vi "Create Bucket.vi"(7 "Request parameters":T1, 8 "error in (no error)":errorcluster, 9 "Bucket":string) -> (0 "error out":errorcluster)   [LabVIEW 2011, in "LV Interface for Amazon S3.lvlib"]
doc: "This operation <B>creates a new bucket</B>. <B>!!! NOTE : For some reason, currently you cannot use the default US Classic region. !!! If you want to use this operation, read through the whole VI Documentation, because the above restriction causes other guidelines you have to follow!</B> To create a bucket, <B>you must register with Amazon S3 and have a valid AWS Access Key ID</B> to authenticate requests. Anonymous requests are never allowed to create buckets. <B>By creating the bucket, you become the bucket owner</B>. When using virtual hosted-style buckets with SSL, the SSL wild card certificate only matches buckets that do not contain periods. To work around this, use HTTP or write your own certificate verification logic. There is no limit to the number of objects that can be stored in a bucket and no variation in performance when using many buckets or just a few. You can store all of your objects in a single bucket or organize them across several buckets. Buckets cannot be nested, meaning buckets cannot be created within buckets. The high availability engineering of Amazon S3 is focused on get, put, list, and delete operations. Because bucket operations work against a centralized, global resource space, it is not appropriate to make bucket create or delete calls on the high availability code path of your application. It is better to create or delete buckets in a separate initialization or setup routine that you run less often. If your application automatically creates buckets, choose a bucket naming scheme that is unlikely to cause naming conflicts. Additionally, make sure your application has logic to choose a different bucket name if a bucket name is already taken."
uses:
  LV Interface for Amazon S3.lvlib
  Typedefs/AMZ_S3_API_PUT Bucket Request Parameters.ctl
  Typedefs/AMZ_S3_ACL.ctl
  Typedefs/AMZ_S3_LocationConstraint.ctl
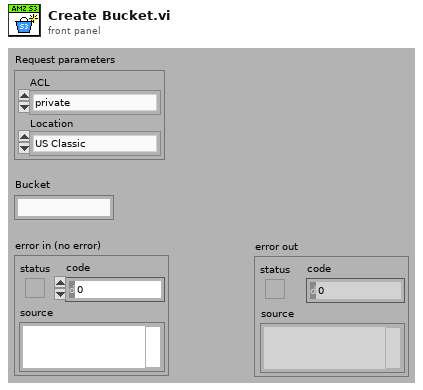
[diagram p1: front panel]
types:
  T1 = typedef "LV Interface for Amazon S3.lvlib/AMZ_S3_API_PUT Bucket Request Parameters.ctl" = cluster{"ACL":T2, "Location":T3}
  T2 = typedef "LV Interface for Amazon S3.lvlib/AMZ_S3_ACL.ctl" = enum16{"private", "public-read", "public-read-write", "authenticated-read", "bucket-owner-read", "bucket-owner-full-control"}
  T3 = typedef "LV Interface for Amazon S3.lvlib/AMZ_S3_LocationConstraint.ctl" = enum16{"US Classic", "EU", "US-West-1", "AP-SouthEast-1"}
  T4 = typedef "LV Interface for Amazon S3.lvlib/AMZ_S3_HTTP Header-Value pair.ctl" = cluster{"Header":string, "Value":string}
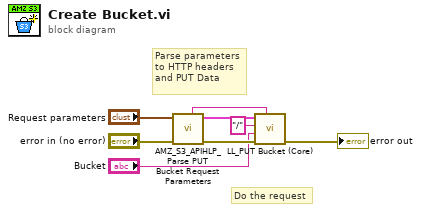
[diagram p0: block diagram]
diagram:
  # "Do the request"
  # "Parse parameters\nto HTTP headers\nand PUT Data"
  n1 = call "AMZ_S3_APIHLP_Parse PUT Bucket Request Parameters.vi"("error in (no error)"="error in (no error)", "PUT Bucket Request parameters"="Request parameters") -> ("error out"=w7:errorcluster, "HTTP Headers"=w6:T4[], "PUT Data"=w5:string)  [unwired: 7 in]
  n2 = call "LL_PUT Bucket (Core).vi"("Data"=w5, "error in (no error)"=w7, "Bucket"="Bucket", "Path and query string"="/", "Headers"=w6) -> ("error out"=→"error out":errorcluster)  [unwired: 3 in, 3 out]
